vi "drive dasar mobile robot.vi"() -> ()   [LabVIEW 2016]
uses:
  <vilib>/Utility/error.llb/Error Cluster From Error Code.vi
  <vilib>/myRIO/Common/Instrument Driver Framework/myRIO v1.0/PWM/vis/myRIO v1.0 Write PWM.vi
  <vilib>/myRIO/Instrument Drivers/Onboard IO/PWM/PWM.lvlib
panel:
  in  "rot ccw":bool
  in  "rot cw":bool
  in  "stop 2":bool
  out "mode":i32
  in  "stop":bool
  in  "Frequency [Hz]":dbl
  in  "dutcy":dbl(slide) scale=0.0..1.0
  in  "maju":bool
  in  "mundur":bool
  in  "kanan":bool
  in  "kiri":bool
  # "1"
  # "4"
  # "3"
  # "2"
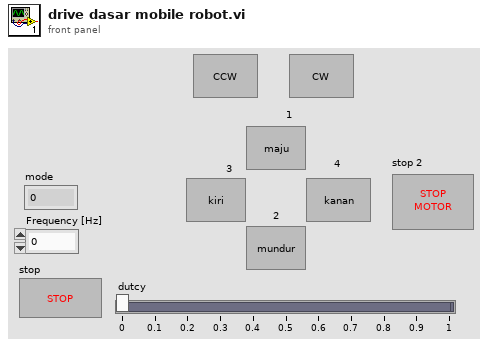
[diagram p1: front panel]
types:
  T1 = enum16{"idle", "maju", "mundur", "kanan", "kiri", "stop motor", "rot cw", "rot ccw"}
  T2 = enum16{"idle", "maju", "mundur", "kanan", "kiri"}
  T3 = typedef "PWM.lvlib/PWM Reference.ctl" = cluster{"myRIO Reference":T4, "PWM Channels Enum":T8, "PWM Configuration":T9}
  T4 = typedef "myRIO Generic Hardware Reference.ctl" = cluster{"myRIO Model":T5, "myRIO Hardware Reference":T6}
  T5 = typedef "Hardware Version Enum.ctl" = enum16{"Unknown", "myRIO-1900", "myRIO-1950", "roboRIO", "NI ELVIS RIO CM"}
  T6 = typedef "myRIO v1.0 Reference.ctl" = cluster{"Generic FPGA Reference":T7, "Allow multiple opens":bool}
  T7 = typedef "Generic FPGA Reference.ctl" = refnum<k20>
  T8 = typedef "PWM Channels Enum.ctl" = enum16{"Not Connected", "C/PWM0", "C/PWM1", "A/PWM0", "A/PWM1", "A/PWM2", "B/PWM0", "B/PWM1", "B/PWM2", "PWM/PWM0", "PWM/PWM1", "PWM/PWM2", "PWM/PWM3", "PWM/PWM4", "PWM/PWM5", "PWM/PWM6", "PWM/PWM7", "PWM/PWM8", "PWM/PWM9"}
  T9 = typedef "PWM.lvlib/PWM Configuration.ctl" = cluster{"Frequency":dbl, "Duty Cycle":dbl}
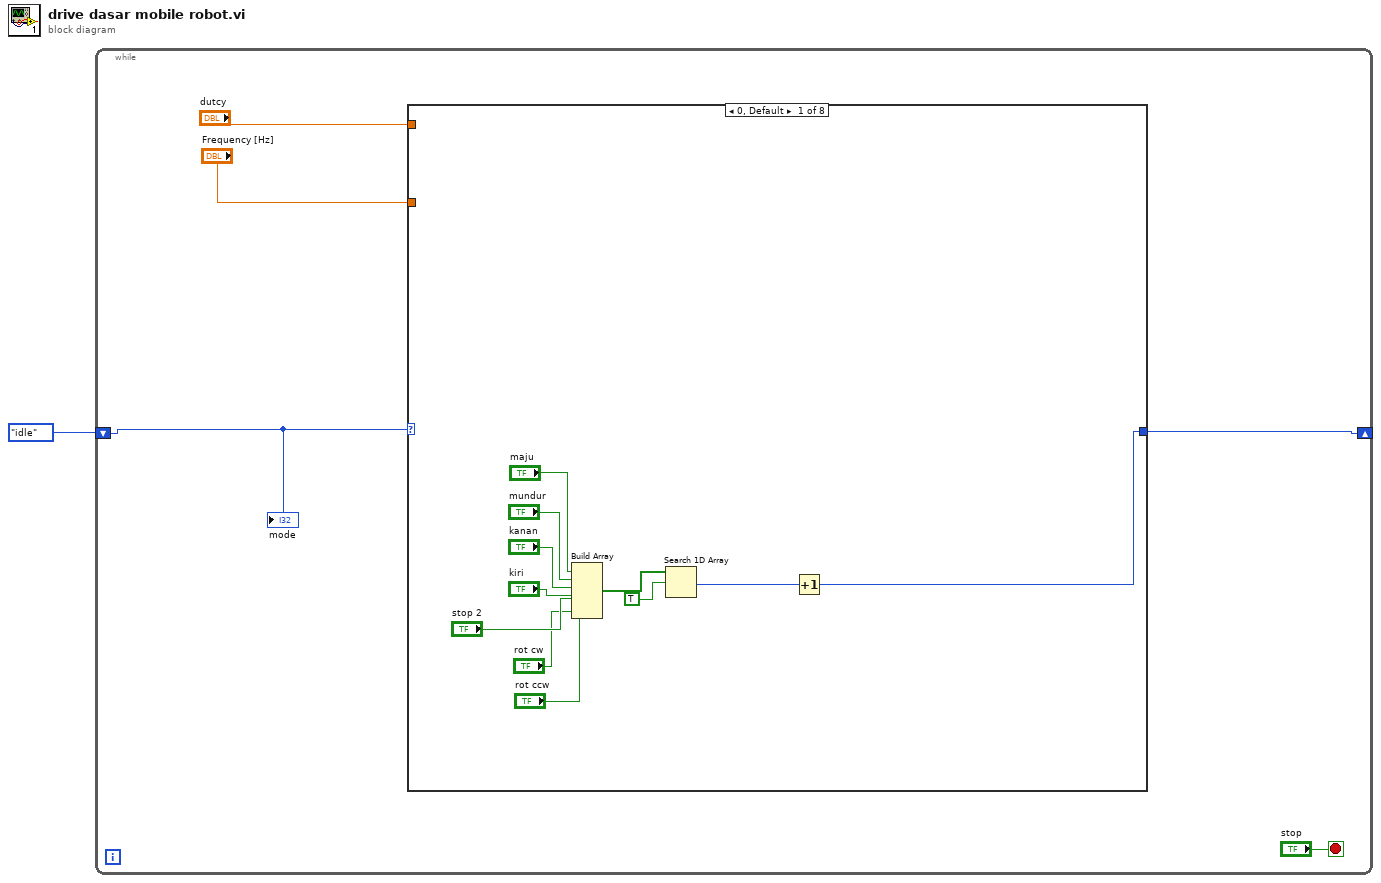
[diagram p0: block diagram]
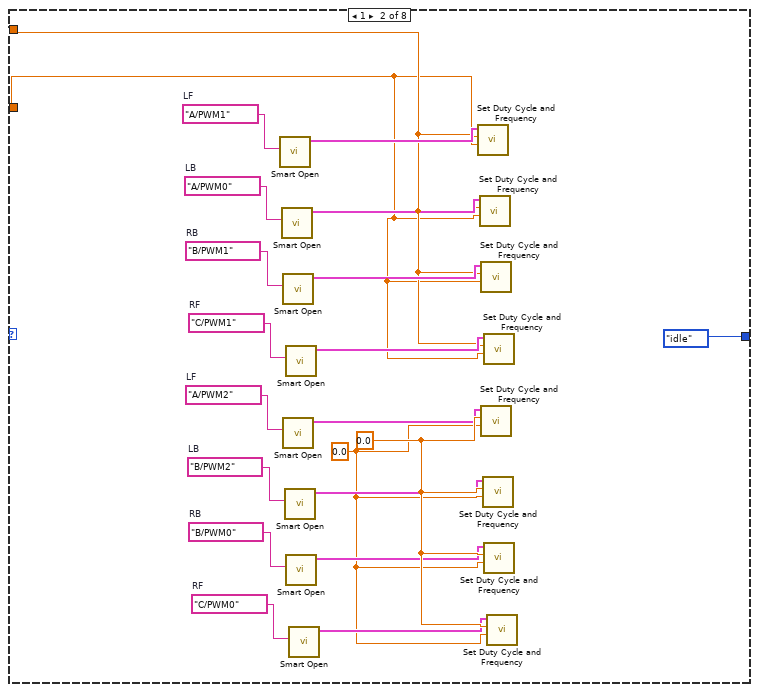
[diagram p2: hidden frame]
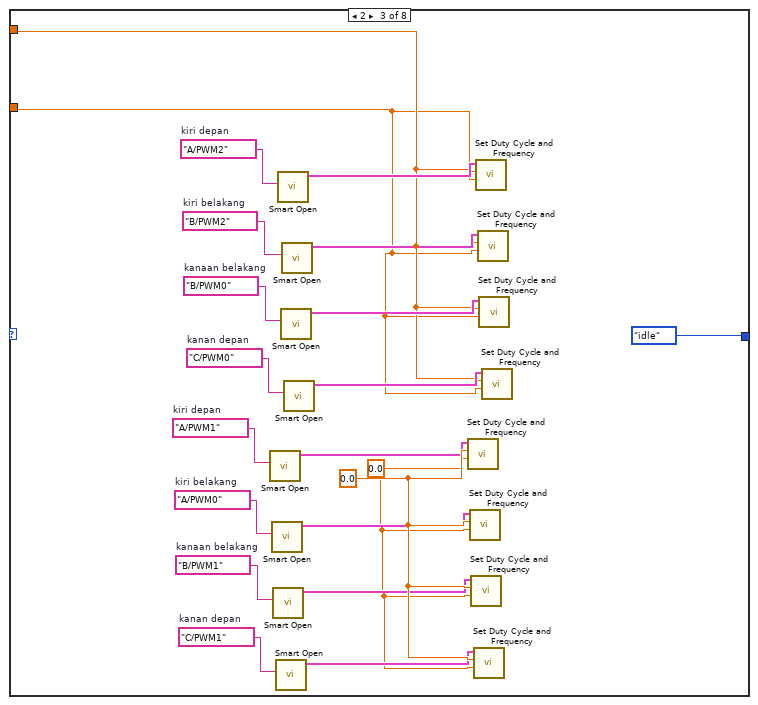
[diagram p3: hidden frame]
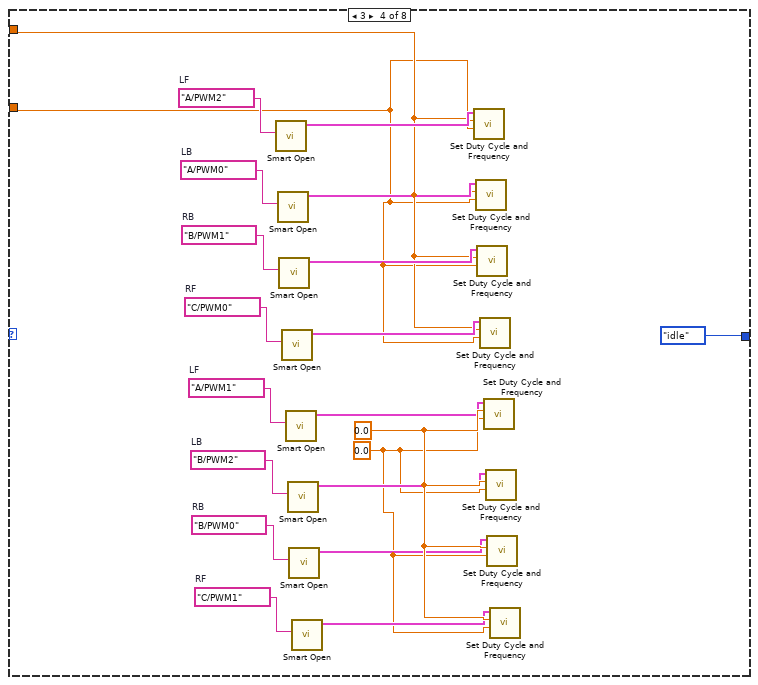
[diagram p4: hidden frame]
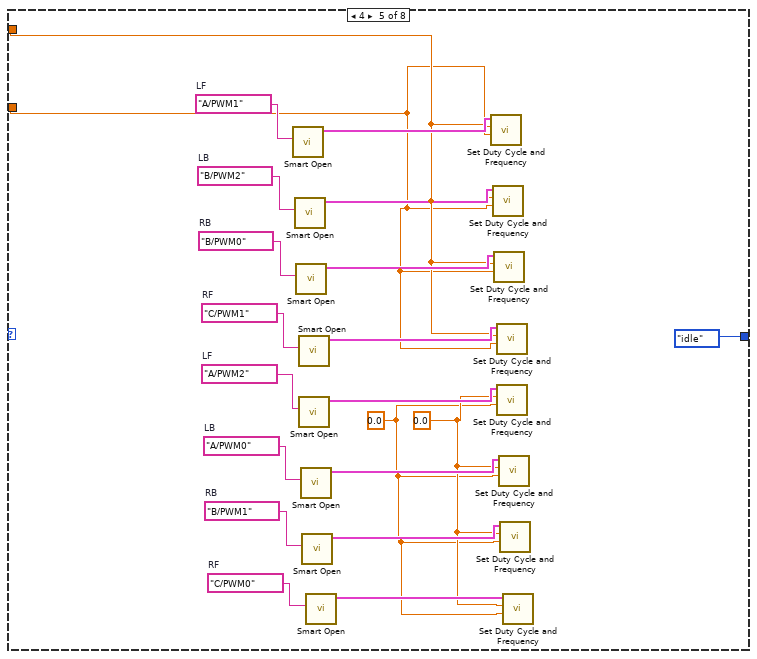
[diagram p5: hidden frame]
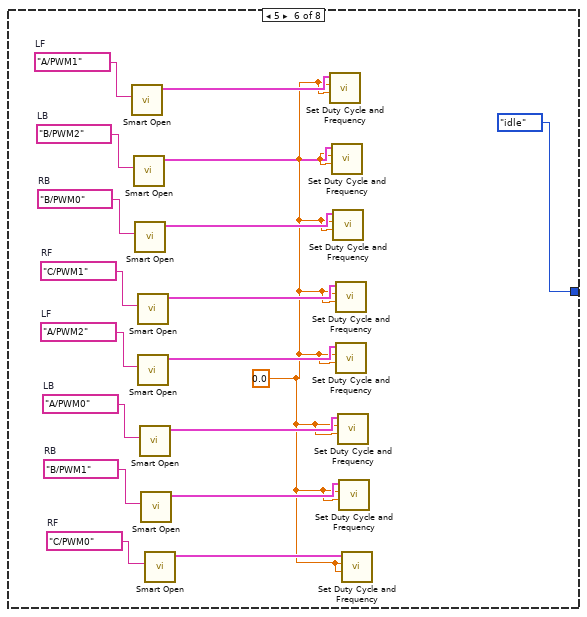
[diagram p6: hidden frame]
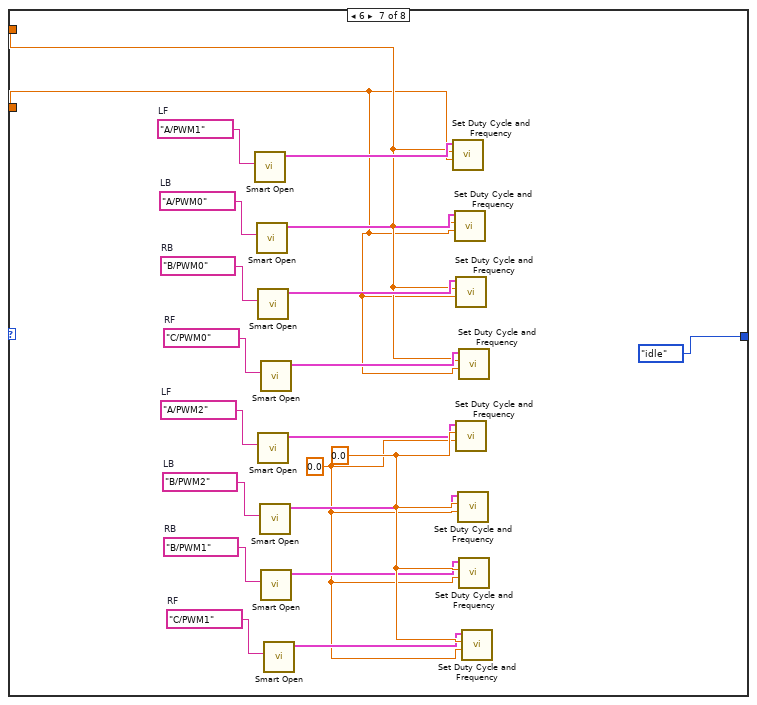
[diagram p7: hidden frame]
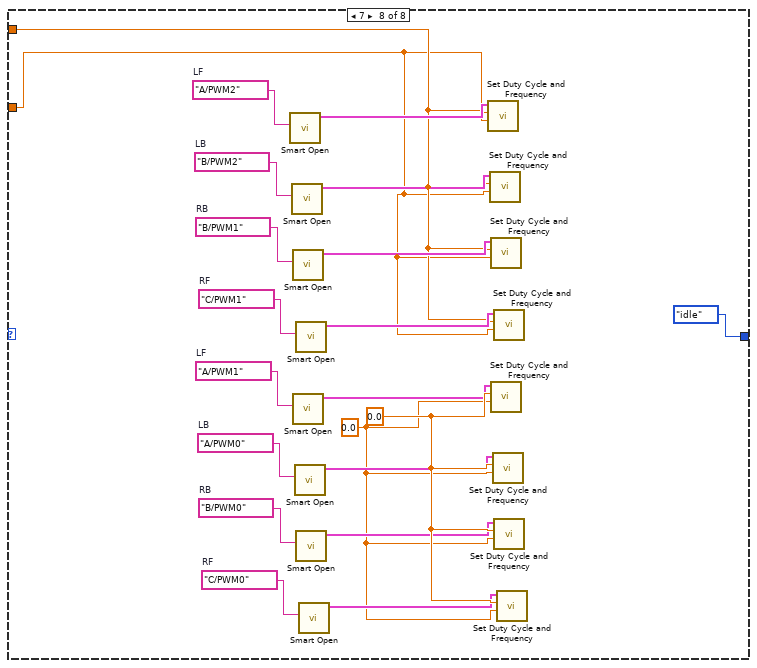
[diagram p8: hidden frame]
diagram:
  n1 = while {
    shift-right: [w2] -> _
    shift-left: T1."idle" -> [w3]
    stop <- "stop" stop-if-true
    n2 = case shown="0, Default" w3 {
      tunnel: "dutcy" -> [_ w30 w51 w72 w93 _ w122 w142]
      tunnel: "Frequency [Hz]" -> [_ w19 w40 w61 w83 _ w121 w141]
      tunnel: [w14 T2."idle" T2."idle" T2."idle" T2."idle" T2."idle" T2."idle" T2."idle"] -> w2
      frame 0, Default {
        n3 = Build Array("maju", "mundur", "kanan", "kiri", "stop 2", "rot cw", "rot ccw") -> (w17:bool[])
        n4 = Search 1D Array(1D array=w17, element=TRUE) -> (index of element=w15:i32)  [unwired: 1 in]
        n5 = Increment(x=w15) -> (x+1=w14:i32)
      }
      frame 1 {
        w18 = 0.0 ("Frequency [Hz]")
        w28 = 0.0 ("Duty Cycle")
        w27 = tag "C/PWM0"  # RF
        w24 = tag "B/PWM0"  # RB
        w23 = tag "B/PWM2"  # LB
        w20 = tag "A/PWM2"  # LF
        w31 = tag "C/PWM1"  # RF
        w34 = tag "B/PWM1"  # RB
        w35 = tag "A/PWM0"  # LB
        w38 = tag "A/PWM1"  # LF
        n6 = call <vilib>:"Smart Open.vi"("Channel Name"=w38) -> ("PWM Ref Out"=w37:T3)  [unwired: 9 in, 1 out]
        n7 = call <vilib>:"Smart Open.vi"("Channel Name"=w35) -> ("PWM Ref Out"=w36:T3)  [unwired: 9 in, 1 out]
        n8 = call <vilib>:"Smart Open.vi"("Channel Name"=w34) -> ("PWM Ref Out"=w33:T3)  [unwired: 9 in, 1 out]
        n9 = call <vilib>:"Smart Open.vi"("Channel Name"=w20) -> ("PWM Ref Out"=w21:T3)  [unwired: 9 in, 1 out]
        n10 = call <vilib>:"Smart Open.vi"("Channel Name"=w23) -> ("PWM Ref Out"=w22:T3)  [unwired: 9 in, 1 out]
        n11 = call <vilib>:"Smart Open.vi"("Channel Name"=w31) -> ("PWM Ref Out"=w32:T3)  [unwired: 9 in, 1 out]
        n12 = call <vilib>:"Smart Open.vi"("Channel Name"=w24) -> ("PWM Ref Out"=w25:T3)  [unwired: 9 in, 1 out]
        n13 = call <vilib>:"Smart Open.vi"("Channel Name"=w27) -> ("PWM Ref Out"=w26:T3)  [unwired: 9 in, 1 out]
        n14 = call <vilib>:"Set Duty Cycle and Frequency.vi"("Frequency [Hz]"=w19, "Duty Cycle"=w30, "PWM Ref In"=w37) -> ()  [unwired: 6 in, 2 out]
        n15 = call <vilib>:"Set Duty Cycle and Frequency.vi"("Frequency [Hz]"=w19, "Duty Cycle"=w30, "PWM Ref In"=w36) -> ()  [unwired: 6 in, 2 out]
        n16 = call <vilib>:"Set Duty Cycle and Frequency.vi"("Frequency [Hz]"=w19, "Duty Cycle"=w30, "PWM Ref In"=w33) -> ()  [unwired: 6 in, 2 out]
        n17 = call <vilib>:"Set Duty Cycle and Frequency.vi"("Frequency [Hz]"=w18, "Duty Cycle"=w28, "PWM Ref In"=w21) -> ()  [unwired: 6 in, 2 out]
        n18 = call <vilib>:"Set Duty Cycle and Frequency.vi"("Frequency [Hz]"=w18, "Duty Cycle"=w28, "PWM Ref In"=w22) -> ()  [unwired: 6 in, 2 out]
        n19 = call <vilib>:"Set Duty Cycle and Frequency.vi"("Frequency [Hz]"=w19, "Duty Cycle"=w30, "PWM Ref In"=w32) -> ()  [unwired: 6 in, 2 out]
        n20 = call <vilib>:"Set Duty Cycle and Frequency.vi"("Frequency [Hz]"=w18, "Duty Cycle"=w28, "PWM Ref In"=w25) -> ()  [unwired: 6 in, 2 out]
        n21 = call <vilib>:"Set Duty Cycle and Frequency.vi"("Frequency [Hz]"=w18, "Duty Cycle"=w28, "PWM Ref In"=w26) -> ()  [unwired: 6 in, 2 out]
      }
      frame 2 {
        w39 = 0.0 ("Frequency [Hz]")
        w49 = 0.0 ("Duty Cycle")
        w48 = tag "C/PWM1"  # kanan depan
        w45 = tag "B/PWM1"  # kanaan belakang
        w44 = tag "A/PWM0"  # kiri belakang
        w41 = tag "A/PWM1"  # kiri depan
        w52 = tag "C/PWM0"  # kanan depan
        w55 = tag "B/PWM0"  # kanaan belakang
        w56 = tag "B/PWM2"  # kiri belakang
        w59 = tag "A/PWM2"  # kiri depan
        n22 = call <vilib>:"Smart Open.vi"("Channel Name"=w41) -> ("PWM Ref Out"=w42:T3)  [unwired: 9 in, 1 out]
        n23 = call <vilib>:"Smart Open.vi"("Channel Name"=w44) -> ("PWM Ref Out"=w43:T3)  [unwired: 9 in, 1 out]
        n24 = call <vilib>:"Smart Open.vi"("Channel Name"=w45) -> ("PWM Ref Out"=w46:T3)  [unwired: 9 in, 1 out]
        n25 = call <vilib>:"Smart Open.vi"("Channel Name"=w48) -> ("PWM Ref Out"=w47:T3)  [unwired: 9 in, 1 out]
        n26 = call <vilib>:"Smart Open.vi"("Channel Name"=w59) -> ("PWM Ref Out"=w58:T3)  [unwired: 9 in, 1 out]
        n27 = call <vilib>:"Smart Open.vi"("Channel Name"=w55) -> ("PWM Ref Out"=w54:T3)  [unwired: 9 in, 1 out]
        n28 = call <vilib>:"Smart Open.vi"("Channel Name"=w56) -> ("PWM Ref Out"=w57:T3)  [unwired: 9 in, 1 out]
        n29 = call <vilib>:"Smart Open.vi"("Channel Name"=w52) -> ("PWM Ref Out"=w53:T3)  [unwired: 9 in, 1 out]
        n30 = call <vilib>:"Set Duty Cycle and Frequency.vi"("Frequency [Hz]"=w39, "Duty Cycle"=w49, "PWM Ref In"=w42) -> ()  [unwired: 6 in, 2 out]
        n31 = call <vilib>:"Set Duty Cycle and Frequency.vi"("Frequency [Hz]"=w39, "Duty Cycle"=w49, "PWM Ref In"=w43) -> ()  [unwired: 6 in, 2 out]
        n32 = call <vilib>:"Set Duty Cycle and Frequency.vi"("Frequency [Hz]"=w39, "Duty Cycle"=w49, "PWM Ref In"=w46) -> ()  [unwired: 6 in, 2 out]
        n33 = call <vilib>:"Set Duty Cycle and Frequency.vi"("Frequency [Hz]"=w39, "Duty Cycle"=w49, "PWM Ref In"=w47) -> ()  [unwired: 6 in, 2 out]
        n34 = call <vilib>:"Set Duty Cycle and Frequency.vi"("Frequency [Hz]"=w40, "Duty Cycle"=w51, "PWM Ref In"=w58) -> ()  [unwired: 6 in, 2 out]
        n35 = call <vilib>:"Set Duty Cycle and Frequency.vi"("Frequency [Hz]"=w40, "Duty Cycle"=w51, "PWM Ref In"=w57) -> ()  [unwired: 6 in, 2 out]
        n36 = call <vilib>:"Set Duty Cycle and Frequency.vi"("Frequency [Hz]"=w40, "Duty Cycle"=w51, "PWM Ref In"=w54) -> ()  [unwired: 6 in, 2 out]
        n37 = call <vilib>:"Set Duty Cycle and Frequency.vi"("Frequency [Hz]"=w40, "Duty Cycle"=w51, "PWM Ref In"=w53) -> ()  [unwired: 6 in, 2 out]
      }
      frame 3 {
        w60 = 0.0 ("Frequency [Hz]")
        w70 = 0.0 ("Duty Cycle")
        w69 = tag "C/PWM1"  # RF
        w66 = tag "B/PWM0"  # RB
        w65 = tag "B/PWM2"  # LB
        w62 = tag "A/PWM1"  # LF
        w73 = tag "C/PWM0"  # RF
        w76 = tag "B/PWM1"  # RB
        w77 = tag "A/PWM0"  # LB
        w80 = tag "A/PWM2"  # LF
        n38 = call <vilib>:"Smart Open.vi"("Channel Name"=w80) -> ("PWM Ref Out"=w79:T3)  [unwired: 9 in, 1 out]
        n39 = call <vilib>:"Smart Open.vi"("Channel Name"=w77) -> ("PWM Ref Out"=w78:T3)  [unwired: 9 in, 1 out]
        n40 = call <vilib>:"Smart Open.vi"("Channel Name"=w76) -> ("PWM Ref Out"=w75:T3)  [unwired: 9 in, 1 out]
        n41 = call <vilib>:"Smart Open.vi"("Channel Name"=w73) -> ("PWM Ref Out"=w74:T3)  [unwired: 9 in, 1 out]
        n42 = call <vilib>:"Smart Open.vi"("Channel Name"=w62) -> ("PWM Ref Out"=w63:T3)  [unwired: 9 in, 1 out]
        n43 = call <vilib>:"Smart Open.vi"("Channel Name"=w65) -> ("PWM Ref Out"=w64:T3)  [unwired: 9 in, 1 out]
        n44 = call <vilib>:"Smart Open.vi"("Channel Name"=w66) -> ("PWM Ref Out"=w67:T3)  [unwired: 9 in, 1 out]
        n45 = call <vilib>:"Smart Open.vi"("Channel Name"=w69) -> ("PWM Ref Out"=w68:T3)  [unwired: 9 in, 1 out]
        n46 = call <vilib>:"Set Duty Cycle and Frequency.vi"("Frequency [Hz]"=w61, "Duty Cycle"=w72, "PWM Ref In"=w79) -> ()  [unwired: 6 in, 2 out]
        n47 = call <vilib>:"Set Duty Cycle and Frequency.vi"("Frequency [Hz]"=w61, "Duty Cycle"=w72, "PWM Ref In"=w78) -> ()  [unwired: 6 in, 2 out]
        n48 = call <vilib>:"Set Duty Cycle and Frequency.vi"("Frequency [Hz]"=w61, "Duty Cycle"=w72, "PWM Ref In"=w75) -> ()  [unwired: 6 in, 2 out]
        n49 = call <vilib>:"Set Duty Cycle and Frequency.vi"("Frequency [Hz]"=w61, "Duty Cycle"=w72, "PWM Ref In"=w74) -> ()  [unwired: 6 in, 2 out]
        n50 = call <vilib>:"Set Duty Cycle and Frequency.vi"("Frequency [Hz]"=w60, "Duty Cycle"=w70, "PWM Ref In"=w63) -> ()  [unwired: 6 in, 2 out]
        n51 = call <vilib>:"Set Duty Cycle and Frequency.vi"("Frequency [Hz]"=w60, "Duty Cycle"=w70, "PWM Ref In"=w64) -> ()  [unwired: 6 in, 2 out]
        n52 = call <vilib>:"Set Duty Cycle and Frequency.vi"("Frequency [Hz]"=w60, "Duty Cycle"=w70, "PWM Ref In"=w67) -> ()  [unwired: 6 in, 2 out]
        n53 = call <vilib>:"Set Duty Cycle and Frequency.vi"("Frequency [Hz]"=w60, "Duty Cycle"=w70, "PWM Ref In"=w68) -> ()  [unwired: 6 in, 2 out]
      }
      frame 4 {
        w81 = 0.0 ("Frequency [Hz]")
        w84 = 0.0 ("Duty Cycle")
        w91 = tag "C/PWM0"  # RF
        w88 = tag "B/PWM1"  # RB
        w87 = tag "A/PWM0"  # LB
        w82 = tag "A/PWM2"  # LF
        w94 = tag "C/PWM1"  # RF
        w97 = tag "B/PWM0"  # RB
        w98 = tag "B/PWM2"  # LB
        w101 = tag "A/PWM1"  # LF
        n54 = call <vilib>:"Smart Open.vi"("Channel Name"=w101) -> ("PWM Ref Out"=w100:T3)  [unwired: 9 in, 1 out]
        n55 = call <vilib>:"Smart Open.vi"("Channel Name"=w98) -> ("PWM Ref Out"=w99:T3)  [unwired: 9 in, 1 out]
        n56 = call <vilib>:"Smart Open.vi"("Channel Name"=w97) -> ("PWM Ref Out"=w96:T3)  [unwired: 9 in, 1 out]
        n57 = call <vilib>:"Smart Open.vi"("Channel Name"=w94) -> ("PWM Ref Out"=w95:T3)  [unwired: 9 in, 1 out]
        n58 = call <vilib>:"Smart Open.vi"("Channel Name"=w82) -> ("PWM Ref Out"=w85:T3)  [unwired: 9 in, 1 out]
        n59 = call <vilib>:"Smart Open.vi"("Channel Name"=w87) -> ("PWM Ref Out"=w86:T3)  [unwired: 9 in, 1 out]
        n60 = call <vilib>:"Smart Open.vi"("Channel Name"=w88) -> ("PWM Ref Out"=w89:T3)  [unwired: 9 in, 1 out]
        n61 = call <vilib>:"Smart Open.vi"("Channel Name"=w91) -> ("PWM Ref Out"=w90:T3)  [unwired: 9 in, 1 out]
        n62 = call <vilib>:"Set Duty Cycle and Frequency.vi"("Frequency [Hz]"=w83, "Duty Cycle"=w93, "PWM Ref In"=w100) -> ()  [unwired: 6 in, 2 out]
        n63 = call <vilib>:"Set Duty Cycle and Frequency.vi"("Frequency [Hz]"=w83, "Duty Cycle"=w93, "PWM Ref In"=w99) -> ()  [unwired: 6 in, 2 out]
        n64 = call <vilib>:"Set Duty Cycle and Frequency.vi"("Frequency [Hz]"=w83, "Duty Cycle"=w93, "PWM Ref In"=w96) -> ()  [unwired: 6 in, 2 out]
        n65 = call <vilib>:"Set Duty Cycle and Frequency.vi"("Frequency [Hz]"=w83, "Duty Cycle"=w93, "PWM Ref In"=w95) -> ()  [unwired: 6 in, 2 out]
        n66 = call <vilib>:"Set Duty Cycle and Frequency.vi"("Frequency [Hz]"=w81, "Duty Cycle"=w84, "PWM Ref In"=w85) -> ()  [unwired: 6 in, 2 out]
        n67 = call <vilib>:"Set Duty Cycle and Frequency.vi"("Frequency [Hz]"=w81, "Duty Cycle"=w84, "PWM Ref In"=w86) -> ()  [unwired: 6 in, 2 out]
        n68 = call <vilib>:"Set Duty Cycle and Frequency.vi"("Frequency [Hz]"=w81, "Duty Cycle"=w84, "PWM Ref In"=w89) -> ()  [unwired: 6 in, 2 out]
        n69 = call <vilib>:"Set Duty Cycle and Frequency.vi"("Frequency [Hz]"=w81, "Duty Cycle"=w84, "PWM Ref In"=w90) -> ()  [unwired: 6 in, 2 out]
      }
      frame 5 {
        w104 = 0.0 ("Duty Cycle")
        w111 = tag "C/PWM0"  # RF
        w108 = tag "B/PWM1"  # RB
        w107 = tag "A/PWM0"  # LB
        w102 = tag "A/PWM2"  # LF
        w112 = tag "C/PWM1"  # RF
        w115 = tag "B/PWM0"  # RB
        w116 = tag "B/PWM2"  # LB
        w119 = tag "A/PWM1"  # LF
        n70 = call <vilib>:"Smart Open.vi"("Channel Name"=w119) -> ("PWM Ref Out"=w118:T3)  [unwired: 9 in, 1 out]
        n71 = call <vilib>:"Smart Open.vi"("Channel Name"=w116) -> ("PWM Ref Out"=w117:T3)  [unwired: 9 in, 1 out]
        n72 = call <vilib>:"Smart Open.vi"("Channel Name"=w115) -> ("PWM Ref Out"=w114:T3)  [unwired: 9 in, 1 out]
        n73 = call <vilib>:"Smart Open.vi"("Channel Name"=w112) -> ("PWM Ref Out"=w113:T3)  [unwired: 9 in, 1 out]
        n74 = call <vilib>:"Smart Open.vi"("Channel Name"=w102) -> ("PWM Ref Out"=w105:T3)  [unwired: 9 in, 1 out]
        n75 = call <vilib>:"Smart Open.vi"("Channel Name"=w107) -> ("PWM Ref Out"=w106:T3)  [unwired: 9 in, 1 out]
        n76 = call <vilib>:"Smart Open.vi"("Channel Name"=w108) -> ("PWM Ref Out"=w109:T3)  [unwired: 9 in, 1 out]
        n77 = call <vilib>:"Smart Open.vi"("Channel Name"=w111) -> ("PWM Ref Out"=w110:T3)  [unwired: 9 in, 1 out]
        n78 = call <vilib>:"Set Duty Cycle and Frequency.vi"("Frequency [Hz]"=w104, "Duty Cycle"=w104, "PWM Ref In"=w118) -> ()  [unwired: 6 in, 2 out]
        n79 = call <vilib>:"Set Duty Cycle and Frequency.vi"("Frequency [Hz]"=w104, "Duty Cycle"=w104, "PWM Ref In"=w117) -> ()  [unwired: 6 in, 2 out]
        n80 = call <vilib>:"Set Duty Cycle and Frequency.vi"("Frequency [Hz]"=w104, "Duty Cycle"=w104, "PWM Ref In"=w114) -> ()  [unwired: 6 in, 2 out]
        n81 = call <vilib>:"Set Duty Cycle and Frequency.vi"("Frequency [Hz]"=w104, "Duty Cycle"=w104, "PWM Ref In"=w113) -> ()  [unwired: 6 in, 2 out]
        n82 = call <vilib>:"Set Duty Cycle and Frequency.vi"("Frequency [Hz]"=w104, "Duty Cycle"=w104, "PWM Ref In"=w105) -> ()  [unwired: 6 in, 2 out]
        n83 = call <vilib>:"Set Duty Cycle and Frequency.vi"("Frequency [Hz]"=w104, "Duty Cycle"=w104, "PWM Ref In"=w106) -> ()  [unwired: 6 in, 2 out]
        n84 = call <vilib>:"Set Duty Cycle and Frequency.vi"("Frequency [Hz]"=w104, "Duty Cycle"=w104, "PWM Ref In"=w109) -> ()  [unwired: 6 in, 2 out]
        n85 = call <vilib>:"Set Duty Cycle and Frequency.vi"("Frequency [Hz]"=w104, "Duty Cycle"=w104, "PWM Ref In"=w110) -> ()  [unwired: 6 in, 2 out]
      }
      frame 6 {
        w123 = 0.0 ("Frequency [Hz]")
        w132 = 0.0 ("Duty Cycle")
        w131 = tag "C/PWM1"  # RF
        w128 = tag "B/PWM1"  # RB
        w127 = tag "B/PWM2"  # LB
        w124 = tag "A/PWM2"  # LF
        w133 = tag "C/PWM0"  # RF
        w136 = tag "B/PWM0"  # RB
        w137 = tag "A/PWM0"  # LB
        w140 = tag "A/PWM1"  # LF
        n86 = call <vilib>:"Smart Open.vi"("Channel Name"=w140) -> ("PWM Ref Out"=w139:T3)  [unwired: 9 in, 1 out]
        n87 = call <vilib>:"Smart Open.vi"("Channel Name"=w137) -> ("PWM Ref Out"=w138:T3)  [unwired: 9 in, 1 out]
        n88 = call <vilib>:"Smart Open.vi"("Channel Name"=w136) -> ("PWM Ref Out"=w135:T3)  [unwired: 9 in, 1 out]
        n89 = call <vilib>:"Smart Open.vi"("Channel Name"=w124) -> ("PWM Ref Out"=w125:T3)  [unwired: 9 in, 1 out]
        n90 = call <vilib>:"Smart Open.vi"("Channel Name"=w127) -> ("PWM Ref Out"=w126:T3)  [unwired: 9 in, 1 out]
        n91 = call <vilib>:"Smart Open.vi"("Channel Name"=w133) -> ("PWM Ref Out"=w134:T3)  [unwired: 9 in, 1 out]
        n92 = call <vilib>:"Smart Open.vi"("Channel Name"=w128) -> ("PWM Ref Out"=w129:T3)  [unwired: 9 in, 1 out]
        n93 = call <vilib>:"Smart Open.vi"("Channel Name"=w131) -> ("PWM Ref Out"=w130:T3)  [unwired: 9 in, 1 out]
        n94 = call <vilib>:"Set Duty Cycle and Frequency.vi"("Frequency [Hz]"=w121, "Duty Cycle"=w122, "PWM Ref In"=w139) -> ()  [unwired: 6 in, 2 out]
        n95 = call <vilib>:"Set Duty Cycle and Frequency.vi"("Frequency [Hz]"=w121, "Duty Cycle"=w122, "PWM Ref In"=w138) -> ()  [unwired: 6 in, 2 out]
        n96 = call <vilib>:"Set Duty Cycle and Frequency.vi"("Frequency [Hz]"=w121, "Duty Cycle"=w122, "PWM Ref In"=w135) -> ()  [unwired: 6 in, 2 out]
        n97 = call <vilib>:"Set Duty Cycle and Frequency.vi"("Frequency [Hz]"=w123, "Duty Cycle"=w132, "PWM Ref In"=w125) -> ()  [unwired: 6 in, 2 out]
        n98 = call <vilib>:"Set Duty Cycle and Frequency.vi"("Frequency [Hz]"=w123, "Duty Cycle"=w132, "PWM Ref In"=w126) -> ()  [unwired: 6 in, 2 out]
        n99 = call <vilib>:"Set Duty Cycle and Frequency.vi"("Frequency [Hz]"=w121, "Duty Cycle"=w122, "PWM Ref In"=w134) -> ()  [unwired: 6 in, 2 out]
        n100 = call <vilib>:"Set Duty Cycle and Frequency.vi"("Frequency [Hz]"=w123, "Duty Cycle"=w132, "PWM Ref In"=w129) -> ()  [unwired: 6 in, 2 out]
        n101 = call <vilib>:"Set Duty Cycle and Frequency.vi"("Frequency [Hz]"=w123, "Duty Cycle"=w132, "PWM Ref In"=w130) -> ()  [unwired: 6 in, 2 out]
      }
      frame 7 {
        w144 = 0.0 ("Frequency [Hz]")
        w153 = 0.0 ("Duty Cycle")
        w152 = tag "C/PWM0"  # RF
        w149 = tag "B/PWM0"  # RB
        w148 = tag "A/PWM0"  # LB
        w145 = tag "A/PWM1"  # LF
        w154 = tag "C/PWM1"  # RF
        w157 = tag "B/PWM1"  # RB
        w158 = tag "B/PWM2"  # LB
        w161 = tag "A/PWM2"  # LF
        n102 = call <vilib>:"Smart Open.vi"("Channel Name"=w161) -> ("PWM Ref Out"=w160:T3)  [unwired: 9 in, 1 out]
        n103 = call <vilib>:"Smart Open.vi"("Channel Name"=w158) -> ("PWM Ref Out"=w159:T3)  [unwired: 9 in, 1 out]
        n104 = call <vilib>:"Smart Open.vi"("Channel Name"=w157) -> ("PWM Ref Out"=w156:T3)  [unwired: 9 in, 1 out]
        n105 = call <vilib>:"Smart Open.vi"("Channel Name"=w145) -> ("PWM Ref Out"=w146:T3)  [unwired: 9 in, 1 out]
        n106 = call <vilib>:"Smart Open.vi"("Channel Name"=w148) -> ("PWM Ref Out"=w147:T3)  [unwired: 9 in, 1 out]
        n107 = call <vilib>:"Smart Open.vi"("Channel Name"=w154) -> ("PWM Ref Out"=w155:T3)  [unwired: 9 in, 1 out]
        n108 = call <vilib>:"Smart Open.vi"("Channel Name"=w149) -> ("PWM Ref Out"=w150:T3)  [unwired: 9 in, 1 out]
        n109 = call <vilib>:"Smart Open.vi"("Channel Name"=w152) -> ("PWM Ref Out"=w151:T3)  [unwired: 9 in, 1 out]
        n110 = call <vilib>:"Set Duty Cycle and Frequency.vi"("Frequency [Hz]"=w141, "Duty Cycle"=w142, "PWM Ref In"=w160) -> ()  [unwired: 6 in, 2 out]
        n111 = call <vilib>:"Set Duty Cycle and Frequency.vi"("Frequency [Hz]"=w141, "Duty Cycle"=w142, "PWM Ref In"=w159) -> ()  [unwired: 6 in, 2 out]
        n112 = call <vilib>:"Set Duty Cycle and Frequency.vi"("Frequency [Hz]"=w141, "Duty Cycle"=w142, "PWM Ref In"=w156) -> ()  [unwired: 6 in, 2 out]
        n113 = call <vilib>:"Set Duty Cycle and Frequency.vi"("Frequency [Hz]"=w144, "Duty Cycle"=w153, "PWM Ref In"=w146) -> ()  [unwired: 6 in, 2 out]
        n114 = call <vilib>:"Set Duty Cycle and Frequency.vi"("Frequency [Hz]"=w144, "Duty Cycle"=w153, "PWM Ref In"=w147) -> ()  [unwired: 6 in, 2 out]
        n115 = call <vilib>:"Set Duty Cycle and Frequency.vi"("Frequency [Hz]"=w141, "Duty Cycle"=w142, "PWM Ref In"=w155) -> ()  [unwired: 6 in, 2 out]
        n116 = call <vilib>:"Set Duty Cycle and Frequency.vi"("Frequency [Hz]"=w144, "Duty Cycle"=w153, "PWM Ref In"=w150) -> ()  [unwired: 6 in, 2 out]
        n117 = call <vilib>:"Set Duty Cycle and Frequency.vi"("Frequency [Hz]"=w144, "Duty Cycle"=w153, "PWM Ref In"=w151) -> ()  [unwired: 6 in, 2 out]
      }
    }
    "mode" <- w3
  }
